vi "CANopen Write SDO.vi"() -> ()   [LabVIEW 2016]
doc: "This example demonstrates how to write CANopen SDO to the device."
uses:
  <vilib>/userdefined/High Color/nirio_resource_hc.ctl
  <vilib>/FPGAPlugInAG/cRIO-9033/niLvFpga_Open_cRIO-9033.vi
  <vilib>/rvi/interface/common/dynamic/niFpgaDynamicAddResources.vi
  <vilib>/CANopenLib/CANOPEN.llb/CANopen Interface Create.vi
  <vilib>/CANopenLib/CANOPEN.llb/CANopen SDO Create.vi
  <vilib>/CANopenLib/CANOPEN.llb/CANopen SDO Write [U32].vi
  <vilib>/CANopenLib/CANOPEN.llb/CANopen SDO Read [U32].vi
  <vilib>/CANopenLib/CANOPEN.llb/CANopen SDO Close.vi
  <vilib>/CANopenLib/CANOPEN.llb/CANopen Interface Close.vi
  <vilib>/FPGAPlugInAG/Dynamic/niLvFpga_Close_Dynamic.vi
  <vilib>/rvi/interface/nirviOpenFPGA/nirviOpenFPGA.xnode
  Users/s163601/Desktop/05-28/FPGA Bitfiles/project_FPGATarget_MainFPGA_S9ZLErdeBuw.lvbitx
  Users/s163601/Desktop/05-28/RT/FPGA/MainFPGA.vi
  <vilib>/rvi/interface/nirviCloseFPGA/nirviCloseFPGA.xnode
panel:
  in  "error in":errorcluster
  out "completion code":u32 format="%.0x"
  in  "node-ID":u8=1 min=1 max=127 step=1
  in  "baud rate":u32(ring)=2 items=["1 Mbit/s"=0, "800 kbit/s"=1, "500 kbit/s"=2, "250 kbit/s"=3, "125 kbit/s"=4, "50 kbit/s"=6, "20 kbit/s"=7, "10 kbit/s"=8]
  in  "CANopen interface":u32(ring) items=["CANopen01", "CANopen02", "CANopen03", "CANopen04", "CANopen05", "CANopen06", "CANopen07", "CANopen08", "CANopen09", "CANopen10", "CANopen11", "CANopen12", "CANopen13", "CANopen14", "CANopen15", "CANopen16", "CANopen17", "CANopen18", "CANopen19", "CANopen20", "CANopen21", "CANopen22", "CANopen23", "CANopen24", "CANopen25", "CANopen26", "CANopen27", "CANopen28", "CANopen29", "CANopen30", "CANopen31", "CANopen32"]
  # "Overview: This example demonstrates how to write CANopen SDO to the device.\nRequirements: Connect CANopen module with a slave device. \nInstructions:\n1. Specify the values of CANopen interface, baud rate of the CANopen interface and node-ID of the slave device.\n2. Run this VI."
  # "Create CANopen interface and SDO object"
  # "Write SDO data"
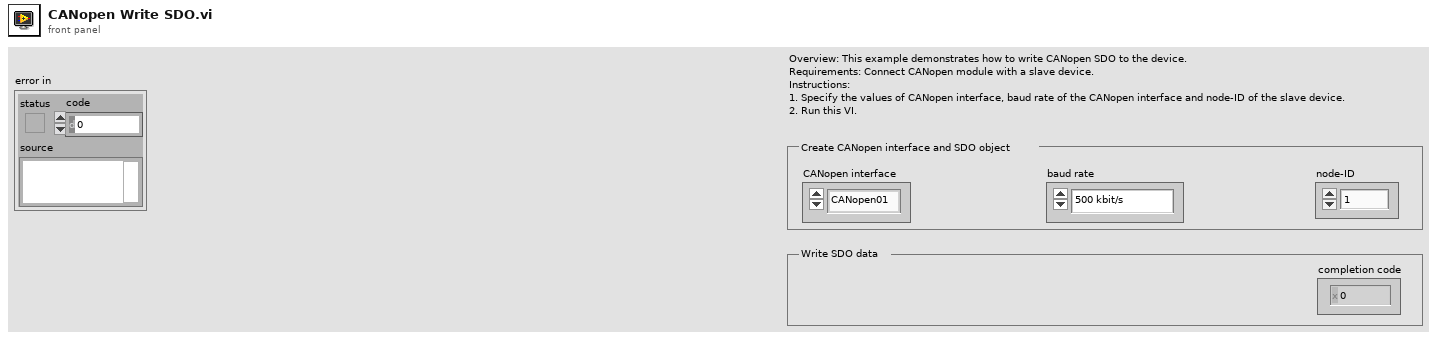
[diagram p1: front panel]
types:
  T1 = typedef "nirio_resource_hc.ctl" = tag
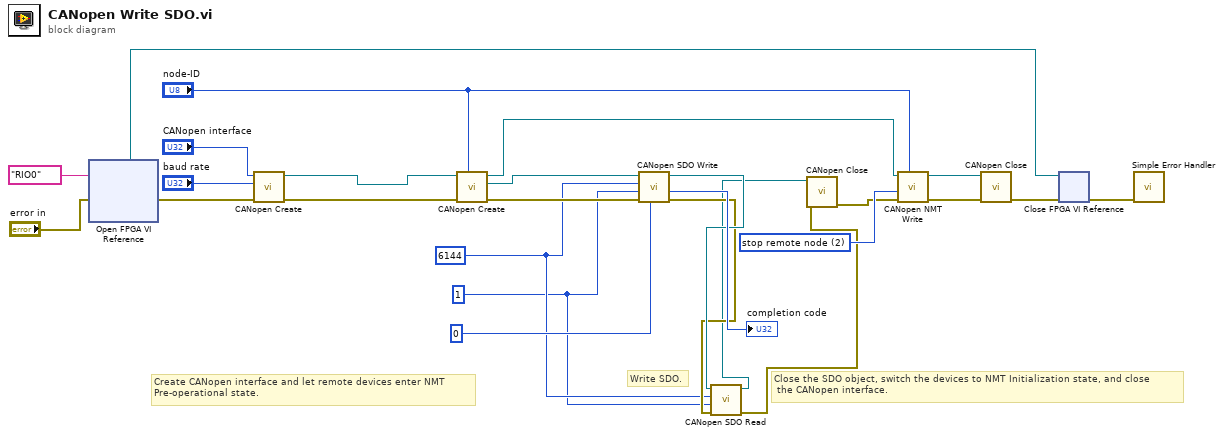
[diagram p0: block diagram]
diagram:
  w1 = u8 1 ("sub-index")
  w2 = u16 6144 ("object index")
  w22 = u16 2 items=["start remote node"=1, "stop remote node"=2, "enter pre-operational"=128, "reset node"=129, "reset communication"=130] ("command")
  # "Create CANopen interface and let remote devices enter NMT\nPre-operational state."
  # "Write SDO."
  # "Close the SDO object, switch the devices to NMT Initialization state, and close\n the CANopen interface."
  n1 = xnode ("Open FPGA VI Reference")("error in"="error in", "resource name"=T1 "RIO0") -> ("FPGA VI Reference Out"=w10:refnum<k20>, "error out"=w13:errorcluster)
  n2 = call-poly <vilib>:"CANopen Create.vi"("error in (no error)"=w13, "baud rate"="baud rate", "interface name"="CANopen interface") -> ("error out"=w7:errorcluster, "interface object out"=w8:refnum<k20>)  [unwired: 7 in]
  n3 = call-poly <vilib>:"CANopen Create.vi"("node-ID"="node-ID", "error in (no error)"=w7, "interface object in"=w8) -> ("error out"=w24:errorcluster, "SDO object out"=w17:refnum<k20>, "interface object out"=w23:refnum<k20>)  [unwired: 6 in]
  n4 = call-poly <vilib>:"CANopen SDO Write.vi"("U32 data"=u8 0 ("write data"), "error in (no error)"=w24, "object sub-index (0)"=w1, "object index"=w2, "SDO object in"=w17) -> ("error out"=w5:errorcluster, "completion code"=→"completion code":u32, "SDO object out"=w6:refnum<k20>)  [unwired: 4 in]
  n5 = call-poly <vilib>:"CANopen SDO Read.vi"("error in (no error)"=w5, "object sub-index (0)"=w1, "object index"=w2, "SDO object in"=w6) -> ("error out"=w3:errorcluster, "SDO object out"=w4:refnum<k20>)  [unwired: 4 in, 2 out]
  n6 = call-poly <vilib>:"CANopen Close.vi"("error in (no error)"=w3, "SDO object in"=w4) -> ("error out"=w20:errorcluster)  [unwired: 9 in]
  n7 = call <vilib>:"CANopen NMT Write.vi"("node-ID (0)"="node-ID", "error in (no error)"=w20, "command"=w22, "interface object in"=w23) -> ("error out"=w19:errorcluster, "interface object out"=w18:refnum<k20>)  [unwired: 6 in]
  n8 = call-poly <vilib>:"CANopen Close.vi"("error in (no error)"=w19, "interface object in"=w18) -> ("error out"=w12:errorcluster)  [unwired: 9 in]
  n9 = xnode "Close FPGA VI Reference"("FPGA VI Reference In"=w10, "error in"=w12) -> ("error out"=w11:errorcluster)
  n10 = call <vilib>:"Simple Error Handler.vi"("error in (no error)"=w11) -> ()  [unwired: 4 in, 5 out]
